vi "Return to Zero.vi"(0 "handle":u32, 1 "Creep":sgl, 2 "Decel":sgl, 3 "ionum":i32, 5 "Axis":i32, 7 "Sramp":sgl, 9 "Accel":sgl, 11 "error in (no error)":errorcluster caption="错误输入（无错误）", 12 "Lspeed":sgl, 13 "Speed":sgl) -> (15 "error out":errorcluster caption="错误输出")   [LabVIEW 2015]
uses:
  zauxdll-2014/zauxdll.lvlib
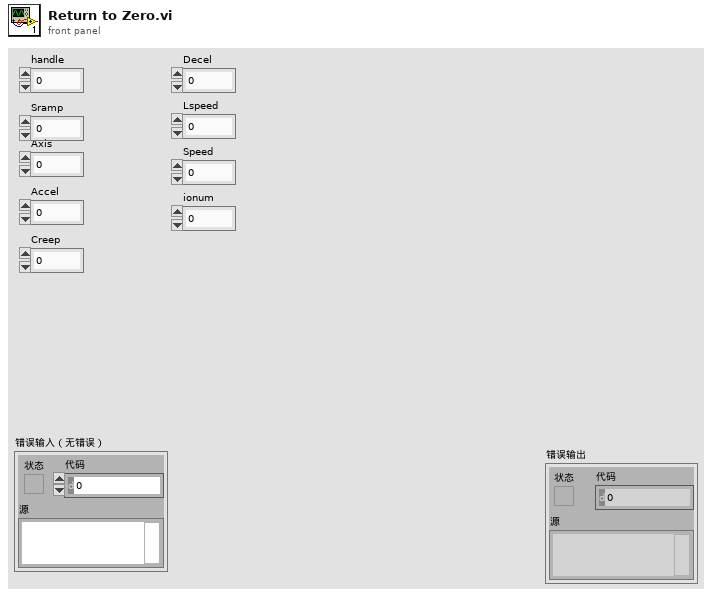
[diagram p1: front panel]
types:
  T1 = cluster{"unsigned byte array[0]":u8, "unsigned byte array[1]":u8, "unsigned byte array[2]":u8, "unsigned byte array[3]":u8, "unsigned byte array[4]":u8, "unsigned byte array[5]":u8, "unsigned byte array[6]":u8, "unsigned byte array[7]":u8, "unsigned byte array[8]":u8}
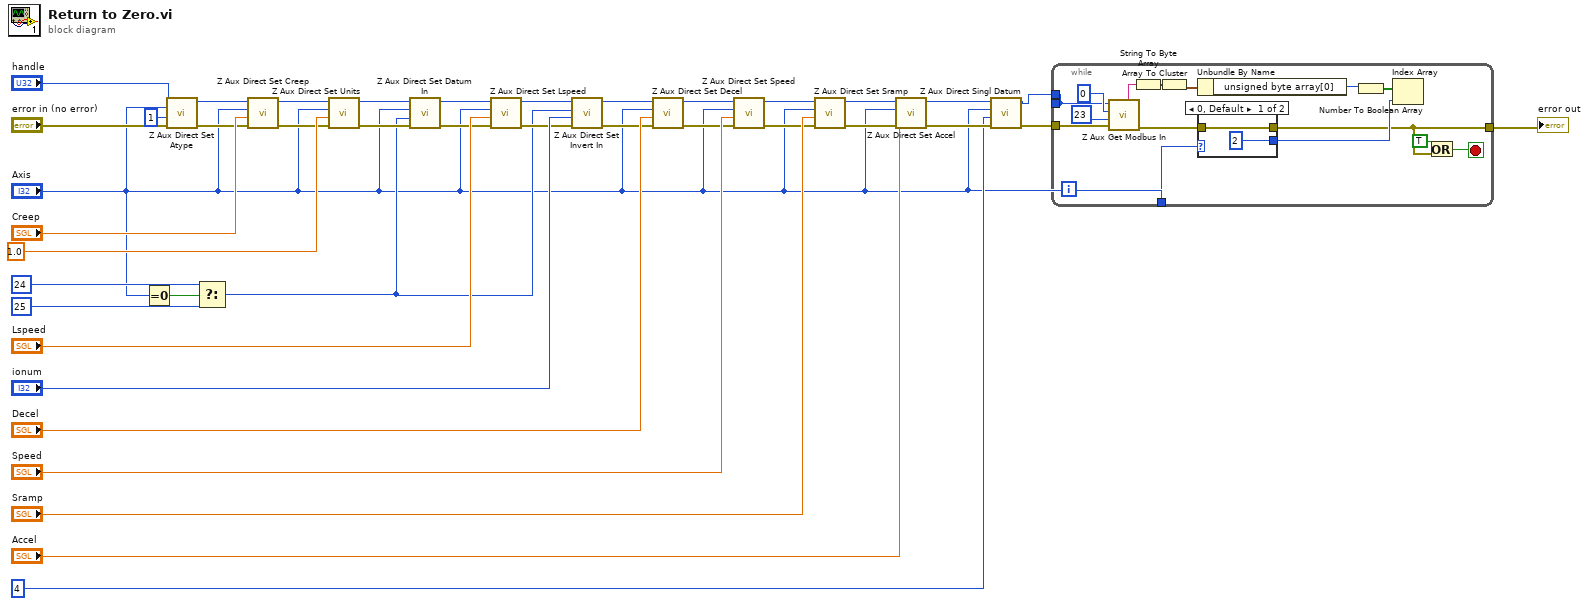
[diagram p0: block diagram]
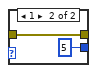
[diagram p2: hidden frame]
diagram:
  n1 = Equal To 0?(x="Axis") -> (x = 0?=w8:bool)
  n2 = call "Z Aux Direct Set Atype.vi"("error in (no error)"="error in (no error)", "iValue"=1, "iaxis"="Axis", "handle"="handle") -> ("error out"=w18:errorcluster, "handle out"=w39:u32)  [unwired: 5 in, 1 out]
  n3 = Select(t=24 ("Org Signal"), s=w8, f=25 ("Org Signal")) -> (s? t:f=w5:i32)
  n4 = call "Z Aux Direct Set Creep.vi"("error in (no error)"=w18, "fValue"="Creep", "iaxis"="Axis", "handle"=w39) -> ("error out"=w17:errorcluster, "handle out"=w38:u32)  [unwired: 5 in, 1 out]
  n5 = call "Z Aux Direct Set Units.vi"("error in (no error)"=w17, "fValue"=sgl 1.0 ("Units"), "iaxis"="Axis", "handle"=w38) -> ("error out"=w16:errorcluster, "handle out"=w37:u32)  [unwired: 5 in, 1 out]
  n6 = call "Z Aux Direct Set Datum In.vi"("error in (no error)"=w16, "iValue"=w5, "iaxis"="Axis", "handle"=w37) -> ("error out"=w15:errorcluster, "handle out"=w36:u32)  [unwired: 5 in, 1 out]
  n7 = call "Z Aux Direct Set Lspeed.vi"("error in (no error)"=w15, "fValue"="Lspeed", "iaxis"="Axis", "handle"=w36) -> ("error out"=w14:errorcluster, "handle out"=w35:u32)  [unwired: 5 in, 1 out]
  n8 = call "Z Aux Direct Set Invert In.vi"("error in (no error)"=w14, "bifInvert"="ionum", "ionum"=w5, "handle"=w35) -> ("error out"=w13:errorcluster, "handle out"=w34:u32)  [unwired: 5 in, 1 out]
  n9 = call "Z Aux Direct Set Decel.vi"("error in (no error)"=w13, "fValue"="Decel", "iaxis"="Axis", "handle"=w34) -> ("error out"=w12:errorcluster, "handle out"=w33:u32)  [unwired: 5 in, 1 out]
  n10 = call "Z Aux Direct Set Speed.vi"("error in (no error)"=w12, "fValue"="Speed", "iaxis"="Axis", "handle"=w33) -> ("error out"=w11:errorcluster, "handle out"=w32:u32)  [unwired: 5 in, 1 out]
  n11 = call "Z Aux Direct Set Sramp.vi"("error in (no error)"=w11, "fValue"="Sramp", "iaxis"="Axis", "handle"=w32) -> ("error out"=w10:errorcluster, "handle out"=w31:u32)  [unwired: 5 in, 1 out]
  n12 = call "Z Aux Direct Set Accel.vi"("error in (no error)"=w10, "fValue"="Accel", "iaxis"="Axis", "handle"=w31) -> ("error out"=w20:errorcluster, "handle out"=w19:u32)  [unwired: 5 in, 1 out]
  n13 = call "Z Aux Direct Singl Datum.vi"("error in (no error)"=w20, "imode"=4, "iaxis"="Axis", "handle"=w19) -> ("error out"=w4:errorcluster, "handle out"=w3:u32)  [unwired: 5 in, 1 out]
  n14 = while {
    tunnel: w4 -> [w55]
    tunnel: [w42] -> _
    tunnel: "Axis" -> [w48]
    tunnel: [w43] -> w1
    tunnel: w3 -> [w42]
    stop <- w44 stop-if-true
    n15 = call "Z Aux Get Modbus In.vi"("error in (no error)"=w55, "ionumend"=23, "ionumfirst"=0, "handle"=w42) -> ("error out"=w49:errorcluster, "pValueList out"=w52:string)  [unwired: 4 in, 2 out]
    n16 = String To Byte Array(string=w52) -> (unsigned byte array=w51:u8[])
    n17 = Array To Cluster(array=w51) -> (cluster=w50:T1)
    n18 = Unbundle By Name(w50) -> ("unsigned byte array[0]"=w46:u8)
    n19 = case shown="0, Default" w48 {
      tunnel: w49 -> [w57 w59]
      tunnel: [w57 w59] -> w43
      tunnel: [2 5] -> w47
      frame 0, Default {
      }
      frame 1 {
      }
    }
    n20 = Number To Boolean Array(number=w46) -> (Boolean array=w45:bool[])
    n21 = Index Array(array=w45, index=w47) -> ()  [unwired: 1 out]
    n22 = Or(x=TRUE, y=w43) -> (x .or. y?=w44:bool)
  }
  "error out" <- w1
